vi "FGV for abort.vi"(11 "write abort":bool) -> (3 "read abort":bool)   [LabVIEW 2023]
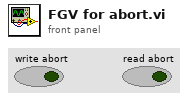
[diagram p1: front panel]
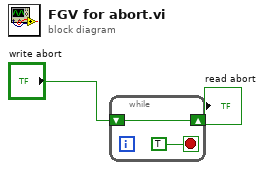
[diagram p0: block diagram]
diagram:
  n1 = while {
    shift-right: [w3] -> w2
    shift-left: "write abort" -> [w3]
    stop <- TRUE stop-if-true
  }
  "read abort" <- w2
